vi "Send Listbox Double Click.vi"(0 "Message Enqueuer in":refnum<class "Message Enqueuer.lvclass">, 1 "Row":i32, 5 "Ctl Refnum":refnum<vi>, 7 "Time":u32, 9 "Coords":T2, 11 "Button":u16, 12 "Mods":cluster{"Double Click":bool, "Menu Key":bool}, 13 "PlatMods":T1) -> (15 "error out":errorcluster)   [LabVIEW 2017, in "ActorEvents.lvlib" / "ListboxDoubleClickMsg.lvclass"]
doc: "<License>\nCopyright © 2017 Composed Systems, LLC | All rights reserved\nwww.composed.io\n\nAuthor: Ethan Stern <ethan.stern@composed.io>\n\nThis software is provided \"AS IS\" WITHOUT WARRANTIES, either express or implied, AND IS FOR EDUCATIONAL PURPOSES ONLY.\n</License>"
uses:
  ListboxDoubleClickMsg.lvclass
  <vilib>/ActorFramework/Message Enqueuer/Message Enqueuer.lvclass
  <vilib>/Utility/miscctls.llb/LVPoint32TypeDef.ctl
  c:/Git/mva-viewable/Source/ActorEvents/IEventAggregator Messages/EventDataMessage/EventDataMessage.lvclass
  ListboxDoubleClickMsg.lvclass/ListboxDoubleClickMsg.ctl
  EventDataMessage/EventDataMessage.lvclass/EventDataMessage.ctl
  <vilib>/ActorFramework/Message Enqueuer/Message Enqueuer.lvclass/Message Enqueuer.ctl
  <vilib>/ActorFramework/Message Enqueuer/Enqueue.vi
  <vilib>/Utility/error.llb/Clear Errors.vi
  EventDataMessage/EventDataMessage.lvclass
  C:/Program Files (x86)/National Instruments/LabVIEW 2017/vi.lib/ActorFramework/Message/Message.lvclass
  <vilib>/ActorFramework/Message Priority Queue/Priority Enqueue.vi
  IEventFilter/IEventFilter.lvclass
panel:
  in  "error in (no error)":errorcluster
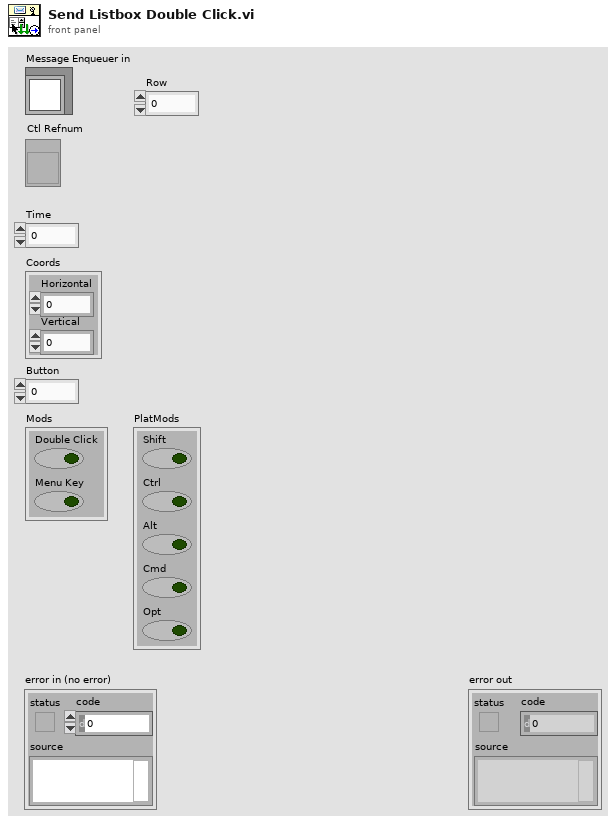
[diagram p1: front panel]
types:
  T1 = cluster{"Shift":bool, "Ctrl":bool, "Alt":bool, "Cmd":bool, "Opt":bool}
  T2 = typedef "LVPoint32TypeDef.ctl" = cluster{"Horizontal":i32, "Vertical":i32}
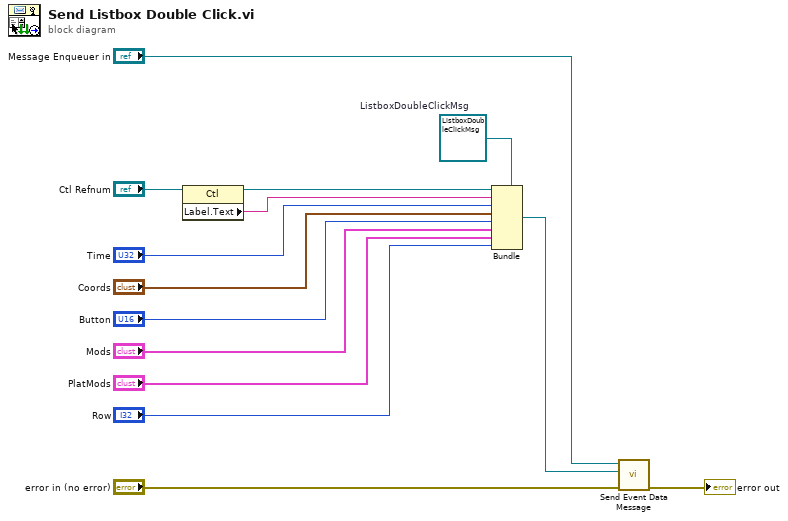
[diagram p0: block diagram]
diagram:
  w14 = refnum<class "ListboxDoubleClickMsg.lvclass"> refnum  # ListboxDoubleClickMsg
  n1 = property class="Ctl"(reference="Ctl Refnum") -> (reference out=w6:refnum<vi>, "Label.Text"=w8:string)  [unwired: 1 in, 1 out]
  n2 = Bundle(cluster=w14, w6, w8, "Time", "Coords", "Button", "Mods", "PlatMods", "Row") -> (w11:refnum<class "ListboxDoubleClickMsg.lvclass">)
  n3 = call "Send Event Data Message.vi"("error in (no error)"="error in (no error)", "EventDataMessage"=w11, "Message Enqueuer in"="Message Enqueuer in") -> ("error out"=→"error out":errorcluster)  [unwired: 7 in, 1 out]
